vi "write csv.vi"(8 "error in (no error)":errorcluster, 10 "file path (dialog if empty)":path, 11 "data log in":refnum<class "data log.lvclass">) -> (0 "error out":errorcluster, 3 "data log out":refnum<class "data log.lvclass">)   [LabVIEW 2025, in "data log.lvclass"]
uses:
  data log.lvclass
  data log.lvclass/data log.ctl
  <vilib>/Utility/file.llb/Write Delimited Spreadsheet (string).vi
panel:
  in  "Save backup (T)":bool=TRUE
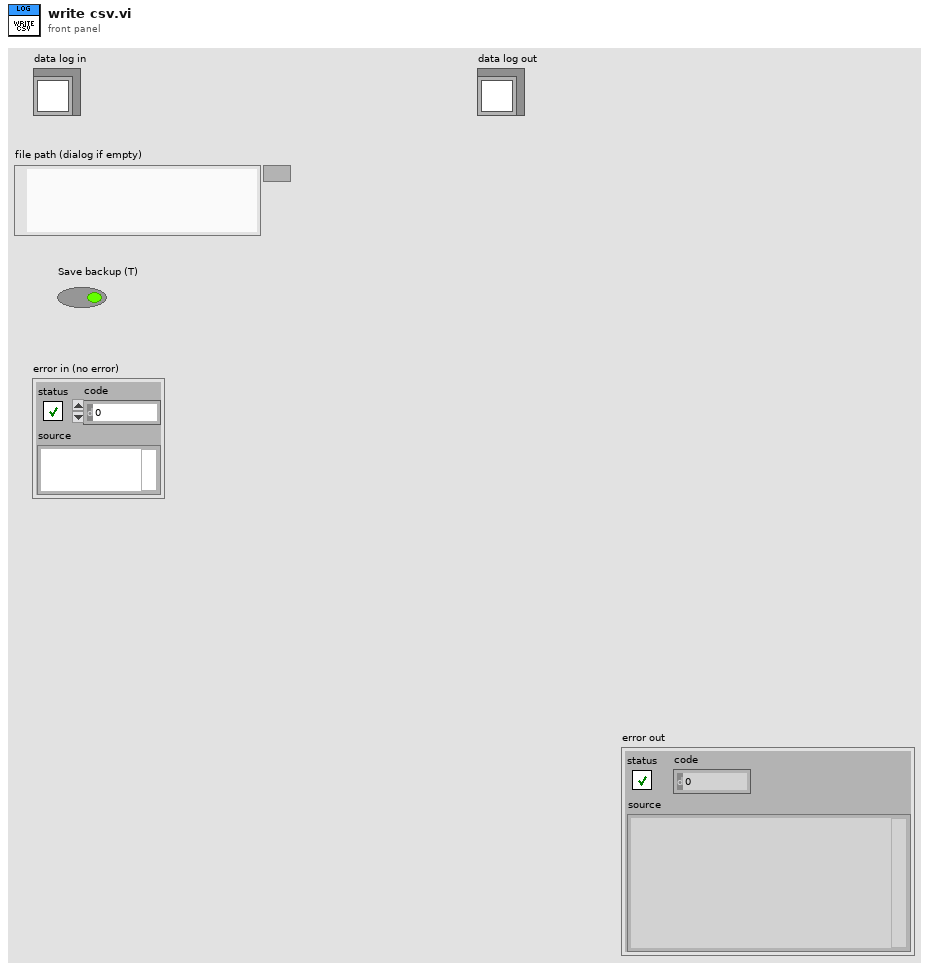
[diagram p1: front panel]
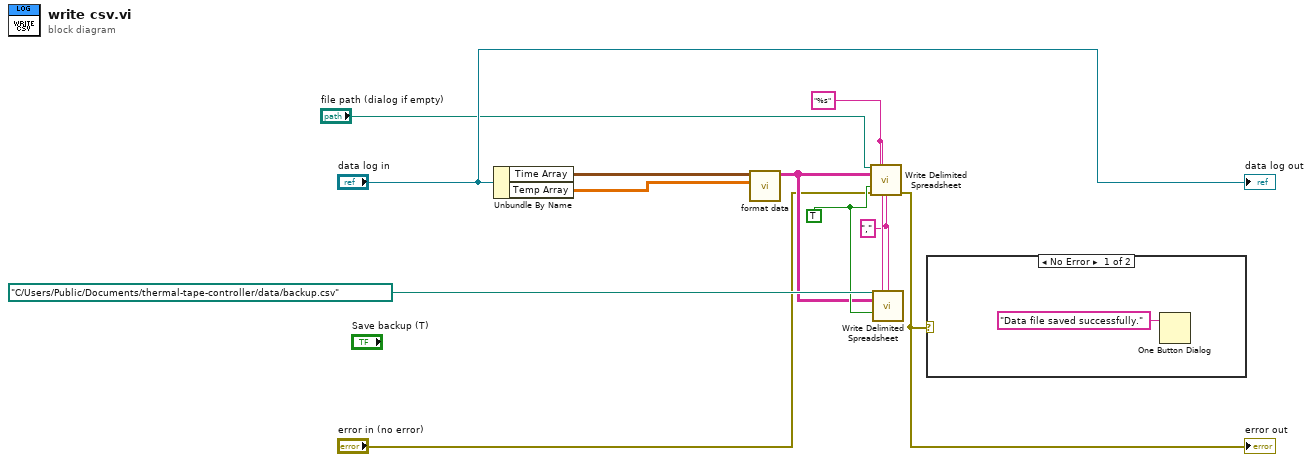
[diagram p0: block diagram]
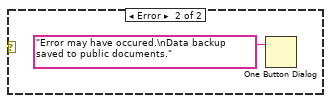
[diagram p2: hidden frame]
diagram:
  w5 = "%s" ("format (%s)")
  w6 = TRUE ("append to file? (new file:F)")
  w3 = "," ("delimiter (\\t)")
  n1 = Unbundle By Name("data log in") -> ("Time Array"=w7:timestamp[][], "Temp Array"=w8:dbl[][])
  n2 = call "format data.vi"("Temp Array"=w8, "Time Array"=w7) -> ("Array"=w4:string[][])  [unwired: 9 in]
  n3 = call-poly <vilib>:"Write Delimited Spreadsheet.vi"("file path (dialog if empty)"="file path (dialog if empty)", "format (%s)"=w5, "2D data"=w4, "append to file? (new file:F)"=w6, "error in (no error)"="error in (no error)", "delimiter (\\t)"=w3) -> ("error out"=w1:errorcluster)  [unwired: 8 in, 1 out]
  "error out" <- w1
  n4 = call-poly <vilib>:"Write Delimited Spreadsheet.vi"("file path (dialog if empty)"=path "C:/Users/Public/Documents/thermal-tape-controller/data/backup.csv", "format (%s)"=w5, "2D data"=w4, "append to file? (new file:F)"=w6, "delimiter (\\t)"=w3) -> ()  [unwired: 9 in, 2 out]
  n5 = case shown="No Error" w1 {
    frame No Error {
      n6 = One Button Dialog(message="Data file saved successfully.") -> ()  [unwired: 1 in, 1 out]
    }
    frame Error {
      n7 = One Button Dialog(message="Error may have occured.\nData backup saved to public documents.") -> ()  [unwired: 1 in, 1 out]
    }
  }
  "data log out" <- "data log in"
